vi "AlliGator Python Plugin Function Offsets.vi"(8 "Error In":errorcluster, 11 "String in":string) -> (0 "Error Out":errorcluster, 2 "Function Offsets":i32[](array[numeric]), 3 "String in (dup)":string, 5 "Script Header":string)   [LabVIEW 2021, in "AlliGator Python Plugins.lvlib"]
doc: "Finds function definition section <B>Offsets</B>.\n\nReturns the script part preceding the first function as <B>Script Header</B>."
uses:
  AlliGator Python Plugins.lvlib
panel:
  # "see the AlliGator License on the block diagram (Ctrl+E or Window:Show Block Diagram)"
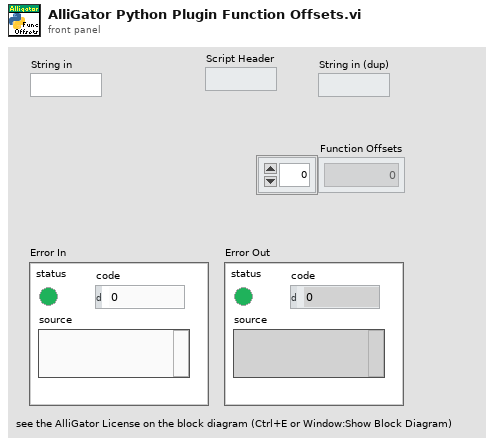
[diagram p1: front panel]
types:
  T1 = enum16{"Native", "Native Command Line", "UNIX", "Macintosh", "DOS"}
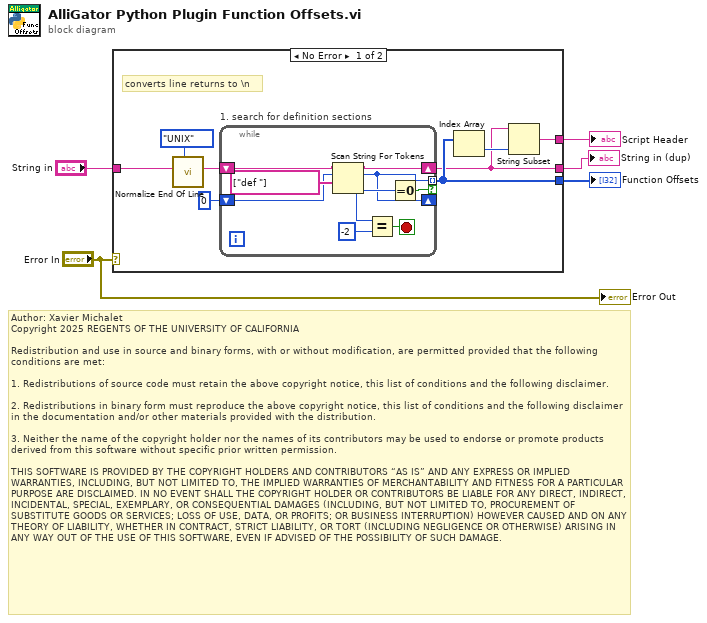
[diagram p0: block diagram]
diagram:
  # "Author: Xavier Michalet\nCopyright 2025 REGENTS OF THE UNIVERSITY OF CALIFORNIA\n\nRedistribution and use in source and binary forms, with or without modification, are permitted provided that the following conditions are met:\n\n1. Redistributions of source code must retain the above copyright notice, this list of conditions and the following disclaimer.\n\n2. Redistributions in binary form must reproduce the above copyright notice, this list of conditions and the following disclaimer in the documentation and/or other materials provided with the distribution.\n\n3. Neither the name of the copyright holder nor the names of its contributors may be used to endorse or promote products derived from this software without specific prior written permission.\n\nTHIS SOFTWARE IS PROVIDED BY THE COPYRIGHT HOLDERS AND CONTRIBUTORS “AS IS” AND ANY EXPRESS OR IMPLIED WARRANTIES, INCLUDING, BUT NOT LIMITED TO, THE IMPLIED WARRANTIES OF MERCHANTABILITY AND FITNESS FOR A PARTICULAR PURPOSE ARE DISCLAIMED. IN NO EVENT SHALL THE COPYRIGHT HOLDER OR CONTRIBUTORS BE LIABLE FOR ANY DIRECT, INDIRECT, INCIDENTAL, SPECIAL, EXEMPLARY, OR CONSEQUENTIAL DAMAGES (INCLUDING, BUT NOT LIMITED TO, PROCUREMENT OF SUBSTITUTE GOODS OR SERVICES; LOSS OF USE, DATA, OR PROFITS; OR BUSINESS INTERRUPTION) HOWEVER CAUSED AND ON ANY THEORY OF LIABILITY, WHETHER IN CONTRACT, STRICT LIABILITY, OR TORT (INCLUDING NEGLIGENCE OR OTHERWISE) ARISING IN ANY WAY OUT OF THE USE OF THIS SOFTWARE, EVEN IF ADVISED OF THE POSSIBILITY OF SUCH DAMAGE."
  n1 = case shown="No Error" "Error In" {
    tunnel: [w9 _] -> w5
    tunnel: [w7 w23] -> w4
    tunnel: "String in" -> [w10 w23]
    tunnel: [w6 _] -> w1
    frame No Error {
      # "converts line returns to \\n"
      n2 = call <vilib>:"Normalize End Of Line.vi"("end of line (Native)"=T1."UNIX", "string in"=w10) -> ("string out"=w12:string)  [unwired: 6 in]
      n3 = while "1. search for definition sections" {
        shift-right: [w21] -> w7
        shift-left: w12 -> [w22]
        tunnel: [w14] -> w9 mode=indexing if=w16
        shift-right: [w14] -> _
        shift-left: 0 ("offset past token") -> [w15]
        stop <- w19 stop-if-true
        n4 = Scan String For Tokens(7:string[] ["def "] ("operators (none)"), 8:w15, 9:w22) -> (0:w17:i32, 2:w14:i32, 3:w21:string)  [unwired: 3 in, 1 out]
        n5 = Equal?(x=w17, y=-2) -> (x = y?=w19:bool)
        n6 = Equal To 0?(x=w17) -> (x = 0?=w16:bool)
      }
      n7 = Index Array(array=w9) -> (element=w8:i32)  [unwired: 1 in]
      n8 = String Subset(string=w7, length (rest)=w8) -> (substring=w6:string)  [unwired: 1 in]
    }
    frame Error {
    }
  }
  "Function Offsets" <- w5
  "String in (dup)" <- w4
  "Script Header" <- w1
  "Error Out" <- "Error In"
